vi "DAQNavi Read (Counter 1D Frequency NChan 1Samp).vi"(8 "error in (no error)":errorcluster, 11 "task in":i32) -> (0 "error out":errorcluster, 2 "data":dbl[](array[numeric]), 3 "task out":i32)   [LabVIEW 2020]
uses:
  DAQNavi_LV.dll
panel:
  in  "timeout":dbl=10.0
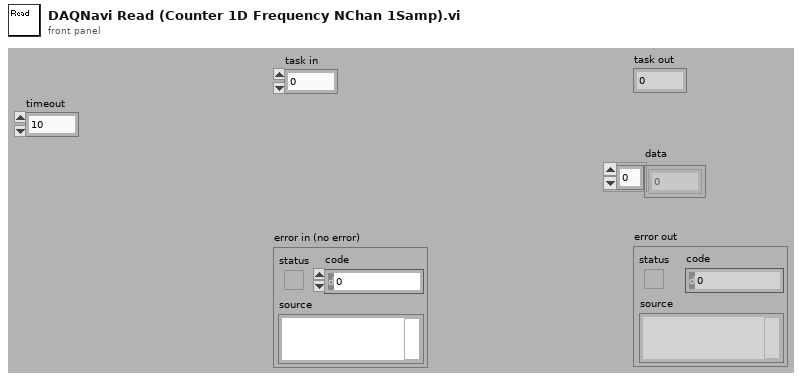
[diagram p1: front panel]
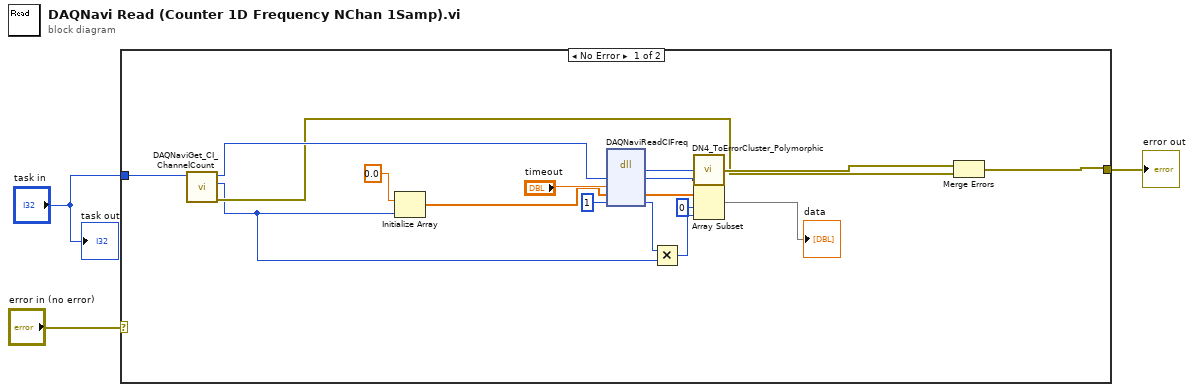
[diagram p0: block diagram]
diagram:
  n1 = case shown="No Error" "error in (no error)" {
    selector: "error in (no error)" -> [_ w21]
    tunnel: "task in" -> [w20 _]
    tunnel: [w9 w21] -> w1
    frame No Error {
      n2 = call "DAQNaviGet_CI_ChannelCount.vi"("task in"=w20) -> ("error out"=w8:errorcluster, "channel count"=w5:i32, "task out"=w12:i32)  [unwired: 1 in, 7 out]
      n3 = Initialize Array(0.0 ("element"), w5) -> (w11:dbl[])
      n4 = dll-call lib="DAQNavi_LV.dll" fn="DAQNaviReadCIFreq"("taskID"=w12, "timeout"="timeout", "freq"=w11, "samples"=u32 1) -> ("return type"=w18:i32, "taskID"=w14:i32, "freq"=w16:dbl[], "samples"=w6:u32)  [unwired: 4 in, 2 out]
      n5 = Multiply(x=w6, y=w5) -> (x*y=w7:u32)
      n6 = call "DN4_ToErrorCluster_Polymorphic.vi"("task id"=w14, "error code"=w18) -> ("error out"=w10:errorcluster)  [unwired: 3 out]
      n7 = Array Subset(array=w16, index=0, length=w7) -> (→"data":dbl[])
      n8 = Merge Errors(w10, w8) -> (w9:errorcluster)
    }
    frame Error {
    }
  }
  "error out" <- w1
  "task out" <- "task in"
